vi "Write irqNumber.vi"(8 "error in (no error)":errorcluster, 10 "irqNumber":i32, 11 "IRQConfig in":refnum<class "IRQConfig.lvclass">) -> (0 "error out":errorcluster, 3 "IRQConfig out":refnum<class "IRQConfig.lvclass">)   [LabVIEW 2013, in "ComponentData.lvlib" / "IRQConfig.lvclass"]
uses:
  <userlib>/Common/Component/Application/RT/ComponentData/ConfigurationHandler/IRQConfig/IRQConfig.lvclass
  <userlib>/Common/Component/Application/RT/ComponentData/ConfigurationHandler/IRQConfig/IRQConfig.lvclass/IRQConfig.ctl
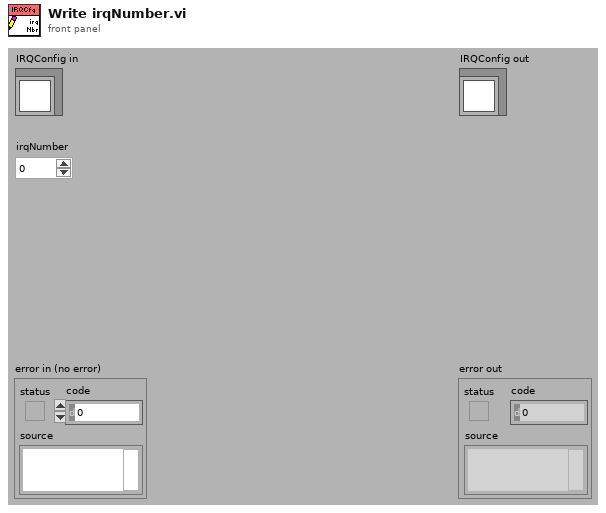
[diagram p1: front panel]
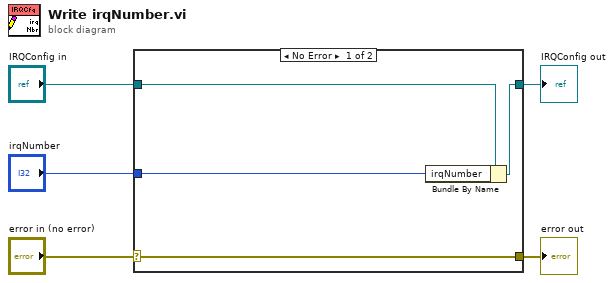
[diagram p0: block diagram]
diagram:
  n1 = case shown="No Error" "error in (no error)" {
    selector: "error in (no error)" -> [w9 w10]
    tunnel: [w9 w10] -> w4
    tunnel: [w7 w11] -> w2
    tunnel: "IRQConfig in" -> [w8 w11]
    tunnel: "irqNumber" -> [w6 _]
    frame No Error {
      n2 = Bundle By Name(cluster=w8, "irqNumber"=w6) -> (w7:refnum<class "IRQConfig.lvclass">)
    }
    frame Error {
    }
  }
  "error out" <- w4
  "IRQConfig out" <- w2
